vi "WPI_DashoardGetDBFileInfo.vi"(9 "Close File":bool, 11 "path":path) -> (0 "error out":errorcluster, 1 "Duration (s)":dbl, 2 "Header":T1, 3 "Byte Stream File out":refnum<file>)   [LabVIEW 2019]
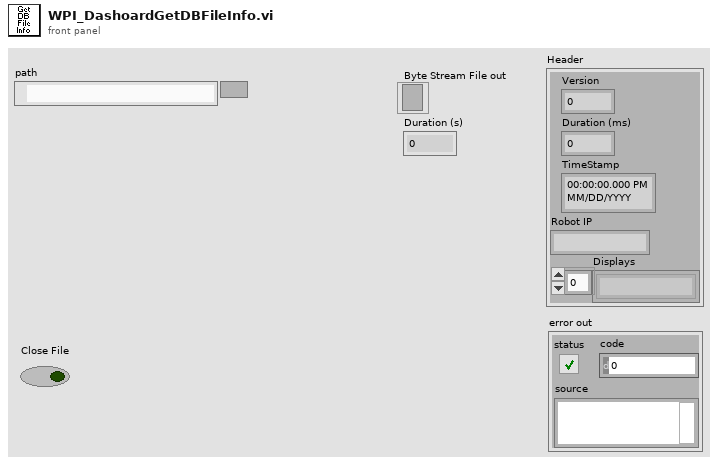
[diagram p1: front panel]
types:
  T1 = cluster{"Version":i32, "Duration (ms)":i32, "TimeStamp":timestamp, "Robot IP":string, "Displays":string[]}
  T2 = cluster{"Version":i32, "Duration (ms)":i32, "TimeStamp":timestamp, "Robot IP":string}
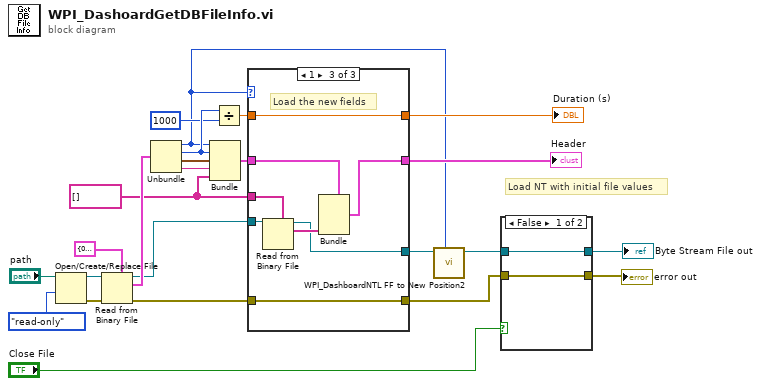
[diagram p0: block diagram]
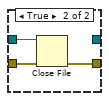
[diagram p2: hidden frame]
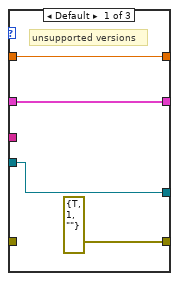
[diagram p3: hidden frame]
diagram:
  w14 = string[] [] ("Displays")
  # "Load NT with initial file values"
  n1 = Open/Create/Replace File(file path (use dialog)="path", access (0:read/write)=enum16{"read/write", "read-only", "write-only"}."read-only") -> (refnum out=w21:refnum<file>, error out=w20:errorcluster)  [unwired: 4 in, 1 out]
  n2 = Read from Binary File(5:T2 {"Version"=0, "Duration (ms)"=0, "TimeStamp"=timestamp(0 s since 1904-01-01), "Robot IP"=""} ("Header"), 8:w20, 11:w21) -> (0:w9:errorcluster, 2:w19:T2, 3:w17:refnum<file>)  [unwired: 3 in, 1 out]
  n3 = Unbundle(w19) -> ("Version"=w3:i32, "Duration (ms)"=w18:i32, "TimeStamp"=w16:timestamp, "Robot IP"=w15:string)
  n4 = Bundle("Version"=w3, "Duration (ms)"=w18, "TimeStamp"=w16, "Robot IP"=w15, "Displays"=w14) -> (w13:T1)  [unwired: 1 in]
  n5 = Divide(x=w18, y=1000) -> (x/y=w10:dbl)
  n6 = case shown="1" w3 {
    tunnel: w17 -> [w25 w29 w40]
    tunnel: [w26 w31 w35] -> w4
    tunnel: w14 -> [_ _ w39]
    tunnel: w13 -> [w28 w32 w37]
    tunnel: [w28 w32 w36] -> w12
    tunnel: w10 -> [w26 w31 w35]
    tunnel: w9 -> [_ w30 w34]
    tunnel: [errorcluster {"status"=TRUE, "code"=1, "source"=""} ("error constant") w30 w34] -> w8
    tunnel: [w25 w29 w33] -> w5
    frame Default {
      # "unsupported versions"
    }
    frame 0 {
    }
    frame 1 {
      # "Load the new fields"
      n7 = Read from Binary File(5:w39, 11:w40) -> (2:w38:string[], 3:w33:refnum<file>)  [unwired: 4 in, 2 out]
      n8 = Bundle(cluster=w37, "Displays"=w38) -> (w36:T1)  [unwired: 4 in]
    }
  }
  "Header" <- w12
  "Duration (s)" <- w4
  n9 = call <vilib>:"WPI_DashboardNTL FF to New Position2.vi"("Version"=w3, "Byte Stream File in"=w5) -> ("Byte Stream File out"=w6:refnum<file>)  [unwired: 6 in, 3 out]
  n10 = case shown="False" "Close File" {
    tunnel: w8 -> [w41 w45]
    tunnel: [w41 w44] -> w7
    tunnel: w6 -> [w42 w43]
    tunnel: [w42 _] -> w2
    frame False {
    }
    frame True {
      n11 = Close File(refnum=w43, error in=w45) -> (error out=w44:errorcluster)  [unwired: 1 out]
    }
  }
  "error out" <- w7
  "Byte Stream File out" <- w2
